vi "Global 1.vi"() -> ()   [LabVIEW 2013]
panel:
  in  "Cycles":i32
  in  "Ping":bool
  in  "OK Button":bool
  out "Time Stamp":timestamp
  out "error out":errorcluster
  in  "Random":dbl
  in  "stop":bool
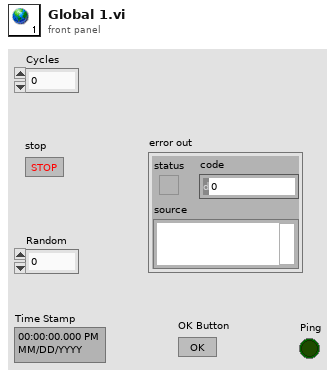
[diagram p1: front panel]
diagram:
